vi "Range_selector.vi"(8 "potential":dbl, 11 "current":dbl) -> (3 "range integer":i32)   [LabVIEW 2022 SP3]
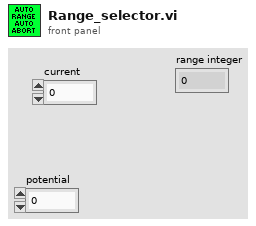
[diagram p1: front panel]
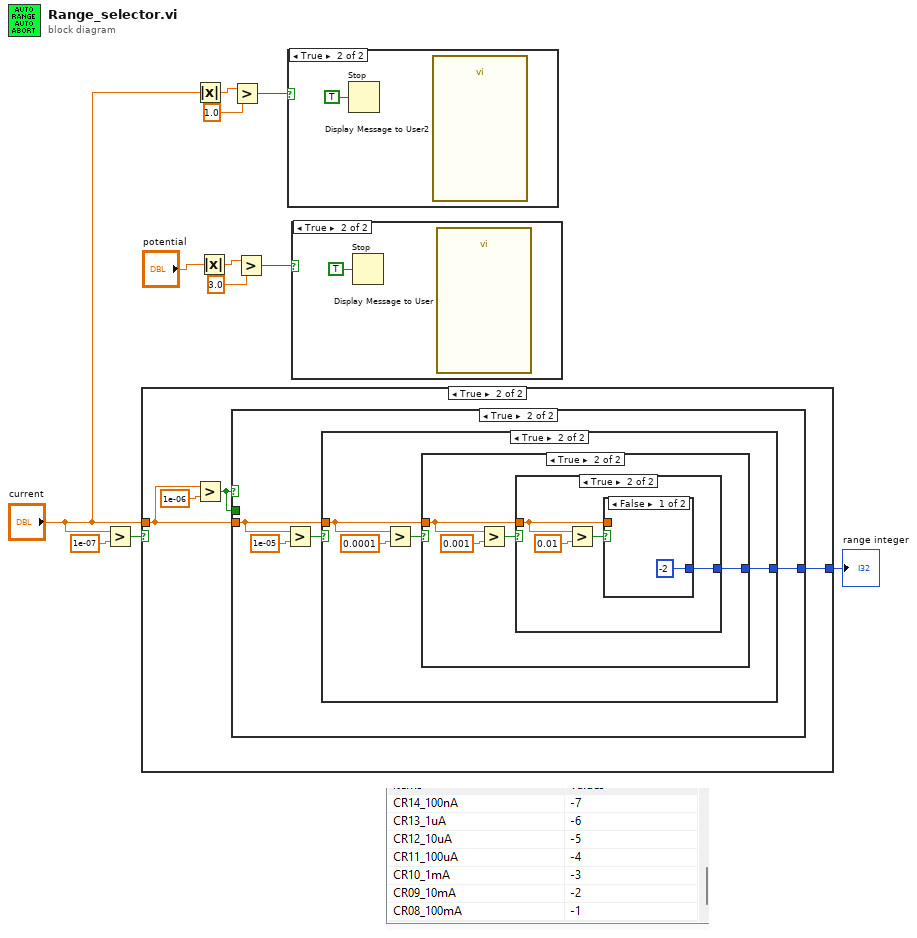
[diagram p0: block diagram]
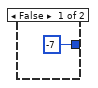
[diagram p4: hidden frame]
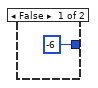
[diagram p5: hidden frame]
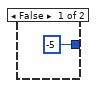
[diagram p6: hidden frame]
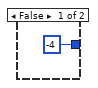
[diagram p7: hidden frame]
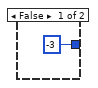
[diagram p8: hidden frame]
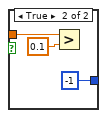
[diagram p9: hidden frame]
diagram:
  n1 = Greater?(x="current", y=1e-07) -> (0:w10:bool)
  n2 = case shown="True" w10 {
    tunnel: "current" -> [_ w15]
    tunnel: [-7 w13] -> w9
    frame False {
    }
    frame True {
      n3 = Greater?(x=w15, y=1e-06) -> (0:w14:bool)
      n4 = case shown="True" w14 {
        tunnel: w14 -> [_ _]
        tunnel: w15 -> [_ w19]
        tunnel: [-6 w18] -> w13
        frame False {
        }
        frame True {
          n5 = Greater?(x=w19, y=1e-05) -> (0:w20:bool)
          n6 = case shown="True" w20 {
            tunnel: w19 -> [_ w24]
            tunnel: [-5 w23] -> w18
            frame False {
            }
            frame True {
              n7 = Greater?(x=w24, y=0.0001) -> (0:w25:bool)
              n8 = case shown="True" w25 {
                tunnel: w24 -> [_ w29]
                tunnel: [-4 w28] -> w23
                frame False {
                }
                frame True {
                  n9 = Greater?(x=w29, y=0.001) -> (0:w30:bool)
                  n10 = case shown="True" w30 {
                    tunnel: w29 -> [_ w34]
                    tunnel: [-3 w33] -> w28
                    frame False {
                    }
                    frame True {
                      n11 = Greater?(x=w34, y=0.01) -> (0:w35:bool)
                      n12 = case shown="False" w35 {
                        tunnel: w34 -> [_ w39]
                        tunnel: [-2 -1] -> w33
                        frame False {
                        }
                        frame True {
                          n13 = Greater?(x=w39, y=0.1) -> ()  [unwired: 1 out]
                        }
                      }
                    }
                  }
                }
              }
            }
          }
        }
      }
    }
  }
  "range integer" <- w9
  n14 = Absolute Value(x="current") -> (abs(x)=w5:dbl)
  n15 = Absolute Value(x="potential") -> (abs(x)=w7:dbl)
  n16 = Greater?(x=w5, y=1.0) -> (0:w1:bool)
  n17 = Greater?(x=w7, y=3.0) -> (0:w2:bool)
  n18 = case shown="True" w1 {
    frame False {
    }
    frame True {
      n19 = Stop(stop? (T)=TRUE) -> ()
      n20 = call "Display Message to User2"() -> ()  [unwired: 10 in, 2 out]
    }
  }
  n21 = case shown="True" w2 {
    frame False {
    }
    frame True {
      n22 = Stop(stop? (T)=TRUE) -> ()
      n23 = call "Display Message to User"() -> ()  [unwired: 10 in, 2 out]
    }
  }
